vi "Get Variables.vi"(8 "error in (no error)":errorcluster, 11 "String Operations in":refnum<class "String Functions.lvclass">) -> (0 "error out":errorcluster, 2 "Variables":variant, 3 "String Operations out":refnum<class "String Functions.lvclass">)   [LabVIEW 2019, in "String Functions.lvclass"]
uses:
  String Functions.lvclass
  String Functions.lvclass/String Functions.ctl
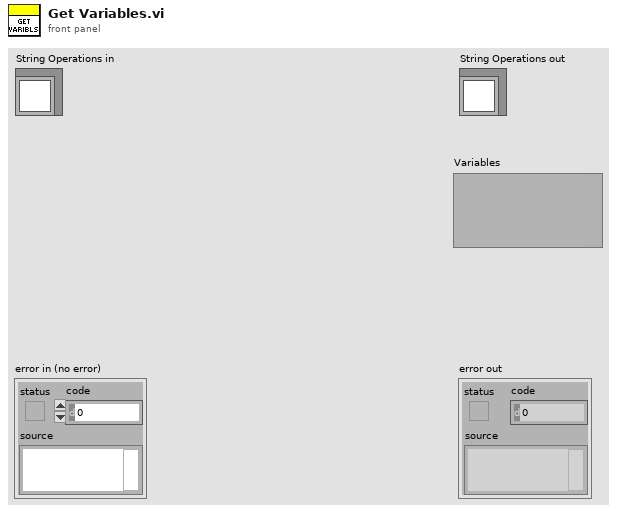
[diagram p1: front panel]
types:
  T1 = typedef "String Functions.lvclass/Variables.ctl" = cluster{"Str1":string, "Str2":string, "offset":i32, "length":i32, "num":dbl}
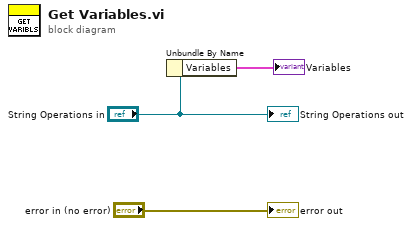
[diagram p0: block diagram]
diagram:
  n1 = Unbundle By Name("String Operations in") -> ("Variables"=→"Variables":T1)
  "error out" <- "error in (no error)"
  "String Operations out" <- "String Operations in"
